vi "Pololu.Mgr - Read Config.vi"(8 "error in (no error)":errorcluster, 10 "Config Folder":path, 11 "PololuCtrl in":refnum<class "PololuCtrl.lvclass">) -> (0 "error out":errorcluster, 2 "Devices":T1[](array[typedef]), 3 "PololuCtrl out":refnum<class "PololuCtrl.lvclass">)   [LabVIEW 2018, in "PololuCtrl.lvclass"]
uses:
  PololuCtrl.lvclass
  SubVIs/Pololu.Device Config.ctl
  SubVIs/Pololu.Device Range Config.ctl
  Utils/Errors/Error.Error Code List.ctl
  PololuCtrl.lvclass/PololuCtrl.ctl
  <vilib>/KATE/Files/File Utils.lvlib
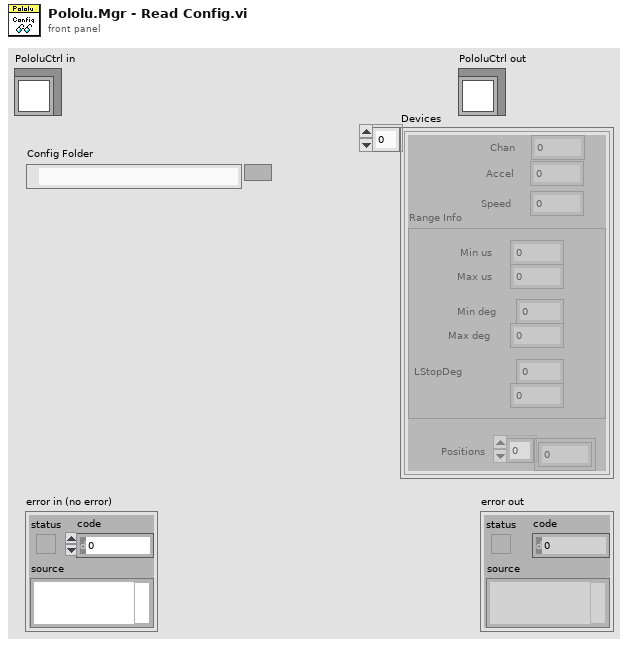
[diagram p1: front panel]
types:
  T1 = typedef "Pololu.Device Config.ctl" = cluster{"Chan":u8, "Accel":u16, "Speed":u16, "Positions":dbl[], "Range Info":T2}
  T2 = typedef "Pololu.Device Range Config.ctl" = cluster{"Min us":dbl, "Max us":dbl, "Min deg":dbl, "Max deg":dbl, "LStopDeg":dbl, "UStopDeg":dbl}
  T3 = typedef "Error.Error Code List.ctl" = i32
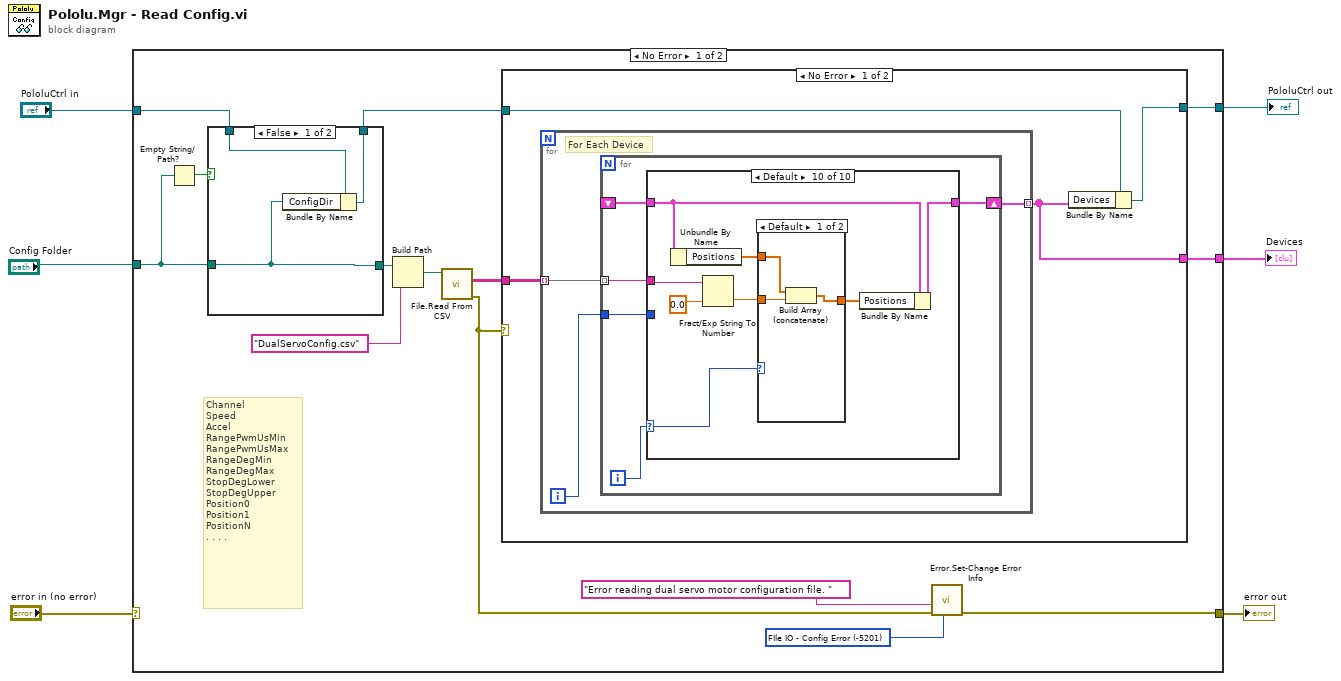
[diagram p0: block diagram]
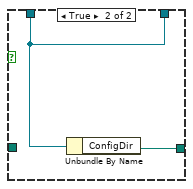
[diagram p2: hidden frame]
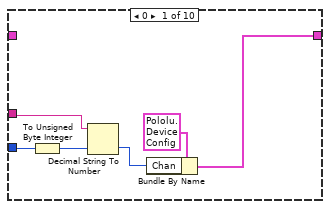
[diagram p3: hidden frame]
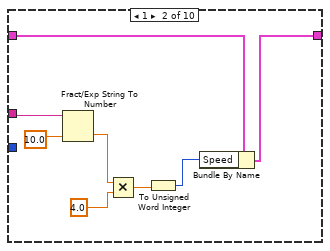
[diagram p4: hidden frame]
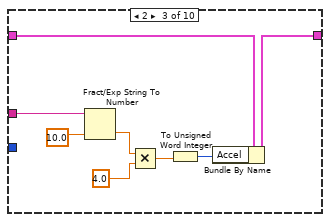
[diagram p5: hidden frame]
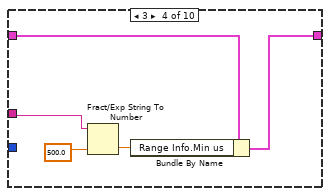
[diagram p6: hidden frame]
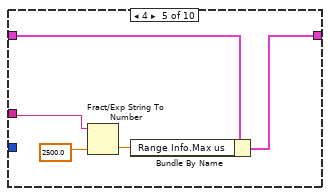
[diagram p7: hidden frame]
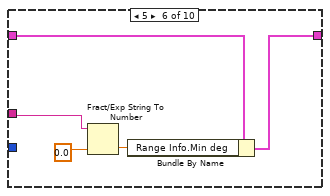
[diagram p8: hidden frame]
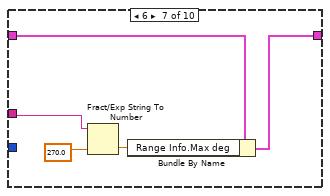
[diagram p9: hidden frame]
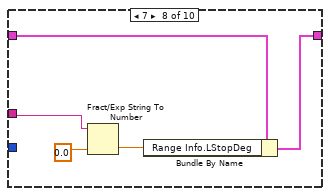
[diagram p10: hidden frame]
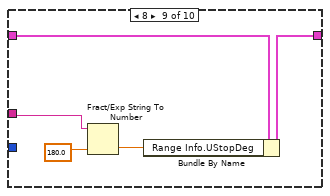
[diagram p11: hidden frame]
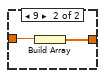
[diagram p12: hidden frame]
diagram:
  n1 = case shown="No Error" "error in (no error)" {
    selector: "error in (no error)" -> [_ w105]
    tunnel: [w19 w105] -> w5
    tunnel: [w14 w104] -> w3
    tunnel: "PololuCtrl in" -> [w11 w104]
    tunnel: "Config Folder" -> [w9 _]
    tunnel: [w7 _] -> w1
    frame No Error {
      w18 = T3 -5201 items=["No Error"=0, "Abort"=-2, "Misc"=-5000, "Fixture Error"=-5100, "File IO - General"=-5200, "FIle IO - Config Error"=-5201, "Instrument - General"=-5300, "Instrument - Serial Com"=-5301, "Instrument - Camera"=-5302, "Instrument - PS"=-5303, "Instrument - Oscilloscope"=-5304, "Instrument - Function Gen"=-5305, "Instrument - Load"=-5306, "Instrument - Meter"=-5307, "Instrument - Power Control"=-5308, "Instrument - Motion"=-5309, "Instrument - RF"=-5310, "System Exe"=-5400, "Image Processing"=-5500, "Communication"=-5600, "Script - Syntax Error"=-6000, "Script - Invalid Name or Param"=-6100, "Script - Timeout"=-6200, "Invalid Data"=-6300, "FW Update Error"=-6500] ("Std Code")
      # "Channel\nSpeed\nAccel\nRangePwmUsMin\nRangePwmUsMax\nRangeDegMin\nRangeDegMax\nStopDegLower\nStopDegUpper\nPosition0\nPosition1\nPositionN\n. . . ."
      n2 = Empty String/Path?(string/path=w9) -> (empty?=w12:bool)
      n3 = case shown="False" w12 {
        tunnel: [w23 w24] -> w10
        tunnel: w9 -> [w22 _]
        tunnel: w11 -> [w21 w24]
        tunnel: [w22 w25] -> w8
        frame False {
          n4 = Bundle By Name(cluster=w21, "ConfigDir"=w22) -> (w23:refnum<class "PololuCtrl.lvclass">)
        }
        frame True {
          n5 = Unbundle By Name(w24) -> ("ConfigDir"=w25:path)
        }
      }
      n6 = Build Path(base path=w8, name or relative path="DualServoConfig.csv") -> (appended path=w13:path)
      n7 = call <vilib>:"File.Read From CSV.vi"("File"=w13) -> ("error out"=w16:errorcluster, "Data"=w15:string[][])  [unwired: 8 in, 1 out]
      n8 = case shown="No Error" w16 {
        tunnel: w15 -> [w29 _]
        tunnel: w10 -> [w28 w103]
        tunnel: [w27 w103] -> w14
        tunnel: [w26 _] -> w7
        frame No Error {
          n9 = for {
            tunnel: w29 -> [w32] mode=indexing
            tunnel: [w31] -> w26 mode=indexing
            i -> [w30]
            # "For Each Device"
            n10 = for {
              tunnel: w32 -> [w36] mode=indexing
              shift-right: [w35] -> w31
              shift-left: _ -> [w37]
              tunnel: w30 -> [w33]
              i -> [w34]
              n11 = case shown="Default" w34 {
                selector: w34 -> [_ _ _ _ _ _ _ _ _ w93]
                tunnel: w37 -> [_ w50 w58 w62 w67 w72 w77 w82 w87 w94]
                tunnel: [w41 w51 w59 w63 w68 w73 w78 w83 w88 w97] -> w35
                tunnel: w36 -> [w38 w48 w52 w60 w65 w70 w75 w80 w85 w95]
                tunnel: w33 -> [w40 _ _ _ _ _ _ _ _ _]
                frame 0 {
                  n12 = To Unsigned Byte Integer(number=w40) -> (unsigned 8bit integer=w39:u8)
                  n13 = Decimal String To Number(string=w38, default (0L)=w39) -> (number=w42:u8)  [unwired: 1 in, 1 out]
                  n14 = Bundle By Name(cluster=T1 {"Chan"=0, "Accel"=10, "Speed"=10, "Positions"=[], "Range Info"={"Min us"=500.0, "Max us"=2500.0, "Min deg"=0.0, "Max deg"=270.0, "LStopDeg"=0.0, "UStopDeg"=270.0}} ("Device"), "Chan"=w42) -> (w41:T1)
                }
                frame 1 {
                  n15 = Fract/Exp String To Number(string=w48, default (0 dbl)=10.0 ("default (0 I32)")) -> (number=w45:dbl)  [unwired: 2 in, 1 out]
                  n16 = Multiply(x=w45, y=4.0) -> (x*y=w47:dbl)
                  n17 = To Unsigned Word Integer(number=w47) -> (unsigned 16bit integer=w44:u16)
                  n18 = Bundle By Name(cluster=w50, "Speed"=w44) -> (w51:T1)
                }
                frame 2 {
                  n19 = Fract/Exp String To Number(string=w52, default (0 dbl)=10.0 ("default (0 I32)")) -> (number=w54:dbl)  [unwired: 2 in, 1 out]
                  n20 = Multiply(x=w54, y=4.0) -> (x*y=w56:dbl)
                  n21 = To Unsigned Word Integer(number=w56) -> (unsigned 16bit integer=w53:u16)
                  n22 = Bundle By Name(cluster=w58, "Accel"=w53) -> (w59:T1)
                }
                frame 3 {
                  n23 = Fract/Exp String To Number(string=w60, default (0 dbl)=500.0 ("default (0 I32)")) -> (number=w64:dbl)  [unwired: 2 in, 1 out]
                  n24 = Bundle By Name(cluster=w62, "Range Info.Min us"=w64) -> (w63:T1)
                }
                frame 4 {
                  n25 = Fract/Exp String To Number(string=w65, default (0 dbl)=2500.0 ("default (0 I32)")) -> (number=w69:dbl)  [unwired: 2 in, 1 out]
                  n26 = Bundle By Name(cluster=w67, "Range Info.Max us"=w69) -> (w68:T1)
                }
                frame 5 {
                  n27 = Fract/Exp String To Number(string=w70, default (0 dbl)=0.0 ("default (0 I32)")) -> (number=w74:dbl)  [unwired: 2 in, 1 out]
                  n28 = Bundle By Name(cluster=w72, "Range Info.Min deg"=w74) -> (w73:T1)
                }
                frame 6 {
                  n29 = Fract/Exp String To Number(string=w75, default (0 dbl)=270.0 ("default (0 I32)")) -> (number=w79:dbl)  [unwired: 2 in, 1 out]
                  n30 = Bundle By Name(cluster=w77, "Range Info.Max deg"=w79) -> (w78:T1)
                }
                frame 7 {
                  n31 = Fract/Exp String To Number(string=w80, default (0 dbl)=0.0 ("default (0 I32)")) -> (number=w84:dbl)  [unwired: 2 in, 1 out]
                  n32 = Bundle By Name(cluster=w82, "Range Info.LStopDeg"=w84) -> (w83:T1)
                }
                frame 8 {
                  n33 = Fract/Exp String To Number(string=w85, default (0 dbl)=180.0 ("default (0 I32)")) -> (number=w89:dbl)  [unwired: 2 in, 1 out]
                  n34 = Bundle By Name(cluster=w87, "Range Info.UStopDeg"=w89) -> (w88:T1)
                }
                frame Default {
                  n35 = Unbundle By Name(w94) -> ("Positions"=w90:dbl[])
                  n36 = Fract/Exp String To Number(string=w95, default (0 dbl)=0.0 ("default (0 I32)")) -> (number=w92:dbl)  [unwired: 2 in, 1 out]
                  n37 = case shown="Default" w93 {
                    tunnel: w92 -> [w99 w102]
                    tunnel: [w98 w101] -> w91
                    tunnel: w90 -> [w100 _]
                    frame Default {
                      n38 = Build Array (concatenate)(w100, w99) -> (w98:dbl[])
                    }
                    frame 9 {
                      n39 = Build Array(w102) -> (w101:dbl[])
                    }
                  }
                  n40 = Bundle By Name(cluster=w94, "Positions"=w91) -> (w97:T1)
                }
              }
            }
          }
          n41 = Bundle By Name(cluster=w28, "Devices"=w26) -> (w27:refnum<class "PololuCtrl.lvclass">)
        }
        frame Error {
        }
      }
      n42 = call "Error.Set-Change Error Info.vi"("Std Code"=w18, "error in"=w16, "Description"="Error reading dual servo motor configuration file. ") -> ("error out"=w19:errorcluster)  [unwired: 8 in]
    }
    frame Error {
    }
  }
  "error out" <- w5
  "PololuCtrl out" <- w3
  "Devices" <- w1
